vi "apiHandle.vi"(8 "error in (no error)":errorcluster, 10 "dataset":cluster{"cmd":string, "data":string}, 11 "User Event in":refnum<user-event>) -> (0 "error out":errorcluster)   [LabVIEW 2018]
uses:
  <vilib>/wsapi/NI_WebServices.lvlib
  <vilib>/Analysis/NI_AALBase.lvlib
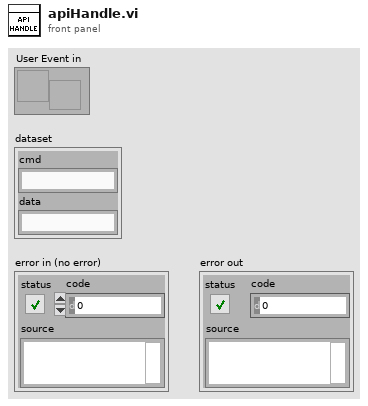
[diagram p1: front panel]
types:
  T1 = typedef "imagedata.ctl" = cluster{"image type":i32, "image depth":i32, "image":u8[], "mask":u8[], "colors":u32[], "Rectangle":cluster{"left":i16, "top":i16, "right":i16, "bottom":i16}}
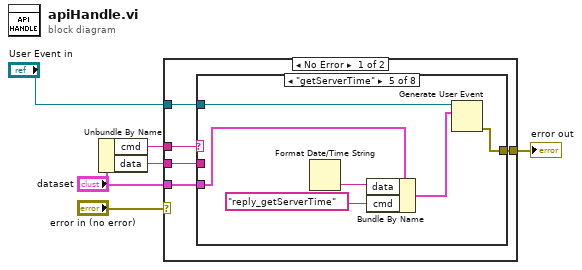
[diagram p0: block diagram]
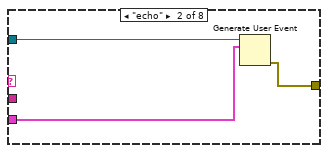
[diagram p3: hidden frame]
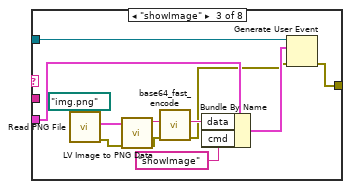
[diagram p4: hidden frame]
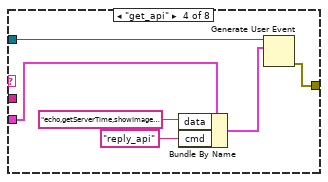
[diagram p5: hidden frame]
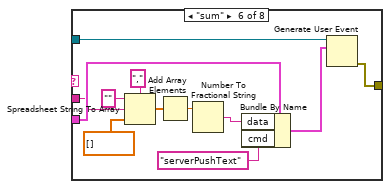
[diagram p6: hidden frame]
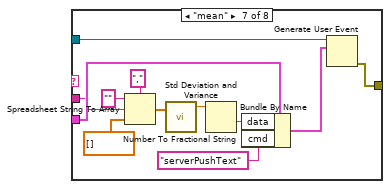
[diagram p7: hidden frame]
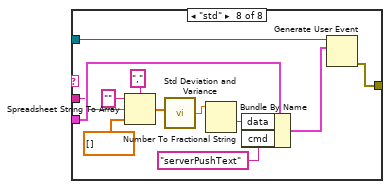
[diagram p8: hidden frame]
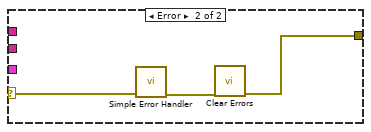
[diagram p9: hidden frame]
diagram:
  n1 = Unbundle By Name("dataset") -> ("cmd"=w3:string, "data"=w4:string)
  n2 = case shown="No Error" "error in (no error)" {
    selector: "error in (no error)" -> [_ w76]
    tunnel: [w7 w77] -> w2
    tunnel: w3 -> [w11 _]
    tunnel: w4 -> [w10 _]
    tunnel: "User Event in" -> [w9 _]
    tunnel: "dataset" -> [w8 _]
    frame No Error {
      n3 = case shown="\"getServerTime\"" w11 {
        tunnel: w10 -> [_ _ _ _ _ w44 w56 w68]
        tunnel: w9 -> [_ w14 w21 w31 w38 w49 w61 w73]
        tunnel: w8 -> [_ w13 w18 w28 w35 w46 w58 w70]
        tunnel: [_ w12 w20 w30 w37 w48 w60 w72] -> w7
        frame "False", Default {
        }
        frame "echo" {
          n4 = Generate User Event(user event=w14, event data cluster=w13) -> (error out=w12:errorcluster)  [unwired: 2 in, 1 out]
        }
        frame "showImage" {
          n5 = call <vilib>:"Read PNG File.vi"("path to PNG file"=path "img.png") -> ("error out"=w17:errorcluster, "image data"=w26:T1)  [unwired: 8 in, 1 out]
          n6 = call <vilib>:"LV Image to PNG Data.vi"("error in (no error)"=w17, "image data"=w26) -> ("error out"=w16:errorcluster, "png data"=w25:string)  [unwired: 8 in]
          n7 = call "base64_fast_encode.vi"("error in (no error)"=w16, "string in (not encoded)"=w25) -> ("error out"=w15:errorcluster, "string out (base64-encoded)"=w23:string)  [unwired: 8 in]
          n8 = Bundle By Name(cluster=w18, "data"=w23, "cmd"="showImage" ("state")) -> (w19:cluster{"cmd":string, "data":string})
          n9 = Generate User Event(user event=w21, event data cluster=w19, error in=w15) -> (error out=w20:errorcluster)  [unwired: 1 in, 1 out]
        }
        frame "get_api" {
          n10 = Bundle By Name(cluster=w28, "data"="echo,getServerTime,showImage,sum,mean,std", "cmd"="reply_api" ("state")) -> (w29:cluster{"cmd":string, "data":string})
          n11 = Generate User Event(user event=w31, event data cluster=w29) -> (error out=w30:errorcluster)  [unwired: 2 in, 1 out]
        }
        frame "getServerTime" {
          n12 = Format Date/Time String() -> (date/time string=w34:string)  [unwired: 3 in]
          n13 = Bundle By Name(cluster=w35, "data"=w34, "cmd"="reply_getServerTime") -> (w36:cluster{"cmd":string, "data":string})
          n14 = Generate User Event(user event=w38, event data cluster=w36) -> (error out=w37:errorcluster)  [unwired: 2 in, 1 out]
        }
        frame "sum" {
          n15 = Spreadsheet String To Array(delimiter (Tab)=",", format string="", spreadsheet string=w44, array type (2D Dbl)=dbl[] []) -> (array=w42:dbl[])
          n16 = Add Array Elements(numeric array=w42) -> (sum=w41:dbl)
          n17 = Number To Fractional String(number=w41) -> (F-format string=w40:string)  [unwired: 3 in]
          n18 = Bundle By Name(cluster=w46, "data"=w40, "cmd"="serverPushText" ("state")) -> (w47:cluster{"cmd":string, "data":string})
          n19 = Generate User Event(user event=w49, event data cluster=w47) -> (error out=w48:errorcluster)  [unwired: 2 in, 1 out]
        }
        frame "mean" {
          n20 = Spreadsheet String To Array(delimiter (Tab)=",", format string="", spreadsheet string=w56, array type (2D Dbl)=dbl[] []) -> (array=w52:dbl[])
          n21 = call <vilib>:"Std Deviation and Variance.vi"("X"=w52) -> ("mean"=w51:dbl)  [unwired: 1 in, 2 out]
          n22 = Number To Fractional String(number=w51) -> (F-format string=w54:string)  [unwired: 3 in]
          n23 = Bundle By Name(cluster=w58, "data"=w54, "cmd"="serverPushText" ("state")) -> (w59:cluster{"cmd":string, "data":string})
          n24 = Generate User Event(user event=w61, event data cluster=w59) -> (error out=w60:errorcluster)  [unwired: 2 in, 1 out]
        }
        frame "std" {
          n25 = Spreadsheet String To Array(delimiter (Tab)=",", format string="", spreadsheet string=w68, array type (2D Dbl)=dbl[] []) -> (array=w64:dbl[])
          n26 = call <vilib>:"Std Deviation and Variance.vi"("X"=w64) -> ("standard deviation"=w63:dbl)  [unwired: 1 in, 2 out]
          n27 = Number To Fractional String(number=w63) -> (F-format string=w66:string)  [unwired: 3 in]
          n28 = Bundle By Name(cluster=w70, "data"=w66, "cmd"="serverPushText" ("state")) -> (w71:cluster{"cmd":string, "data":string})
          n29 = Generate User Event(user event=w73, event data cluster=w71) -> (error out=w72:errorcluster)  [unwired: 2 in, 1 out]
        }
      }
    }
    frame Error {
      n30 = call <vilib>:"Simple Error Handler.vi"("error in (no error)"=w76) -> ("error out"=w75:errorcluster)  [unwired: 4 in, 4 out]
      n31 = call <vilib>:"Clear Errors.vi"("error in (no error)"=w75) -> ("error out"=w77:errorcluster)  [unwired: 5 in, 1 out]
    }
  }
  "error out" <- w2
